vi "启动参数设置.vi"() -> ()   [LabVIEW 2016, in "斯坦道总磷总氮.lvlib"]
uses:
  <vilib>/Utility/miscctls.llb/LVPointTypeDef.ctl
  Listbox/Implementations/Listbox/Listbox.lvclass
  <vilib>/Utility/miscctls.llb/LVStringsAndValuesArrayTypeDef_U16.ctl
  Listbox/Implementations/Listbox Item/Listbox Item.lvclass
  Listbox/Implementations/Listbox/Listbox.lvclass/Listbox.ctl
  Listbox/Implementations/Listbox Item/Listbox Item.lvclass/Listbox Item.ctl
  <vilib>/Utility/config.llb/NI_LVConfig.lvlib
panel:
  in  "Move to Left":bool
  in  "Move to Right":bool
  in  "启用的参数":i32(listbox)
  in  "参数列表":i32(listbox)
  in  "取消":bool
  in  "确认":bool
  # "请选择启动参数"
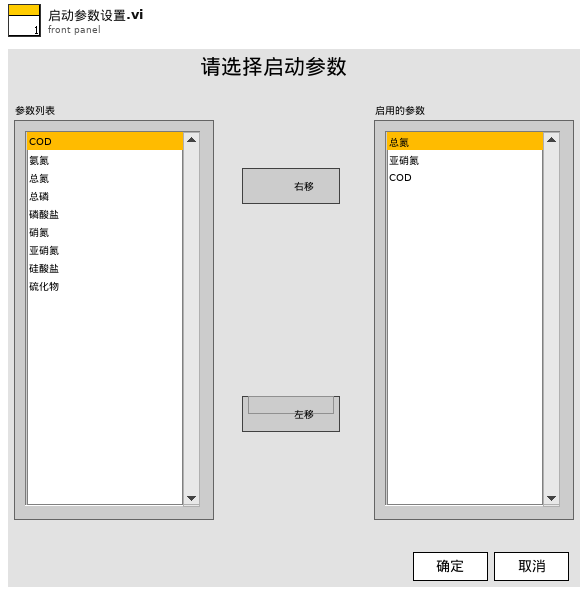
[diagram p1: front panel]
types:
  T1 = typedef "LVStringsAndValuesArrayTypeDef_U16.ctl" = cluster{"String":string, "Value":u16}[]
  T2 = typedef "LVPointTypeDef.ctl" = cluster{"Horizontal":i16, "Vertical":i16}
  T3 = typedef "NI_LVConfig.lvlib/Config Data RefNum.ctl" = refnum<k1>
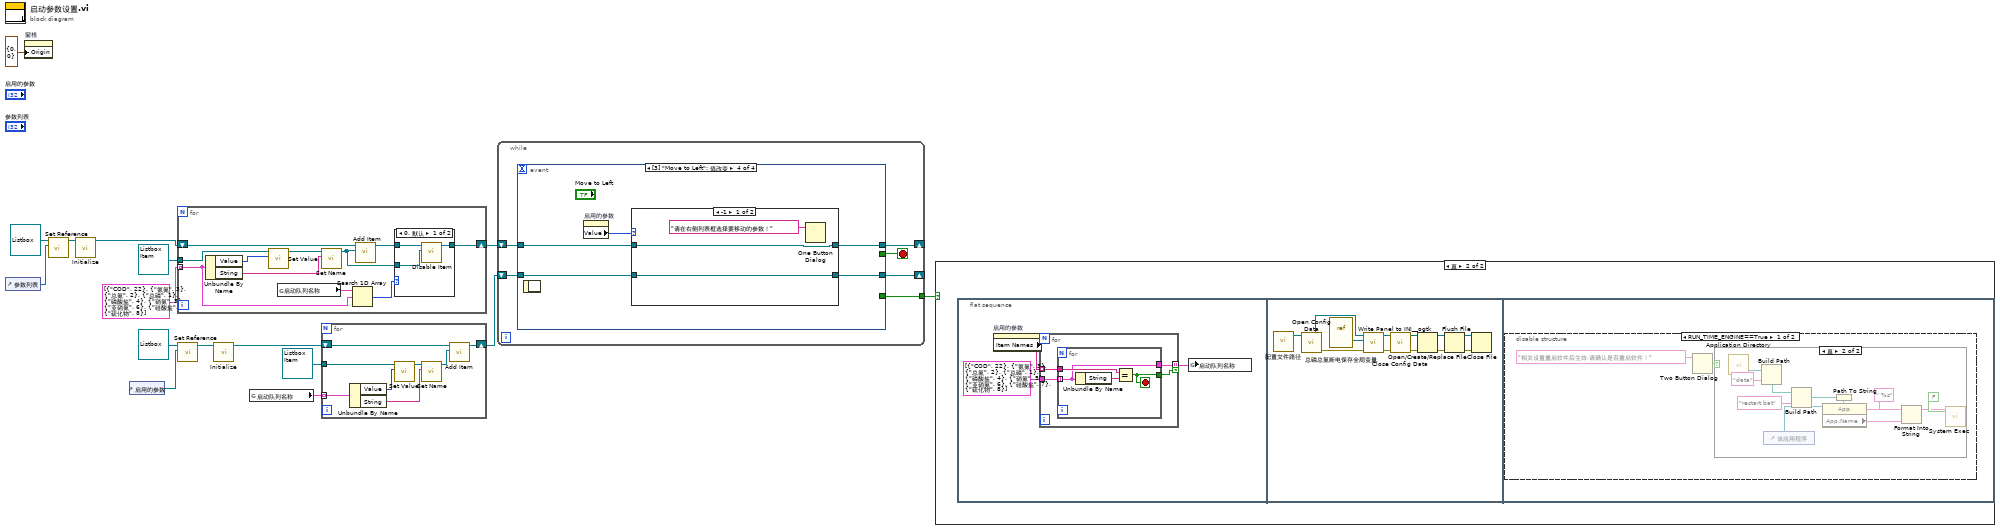
[diagram p0: block diagram]
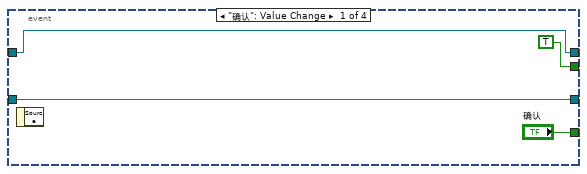
[diagram p2: hidden frame]
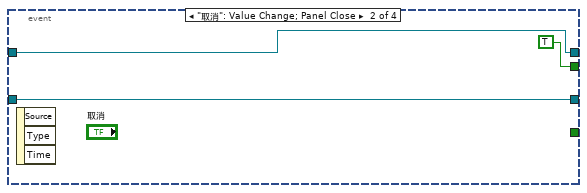
[diagram p3: hidden frame]
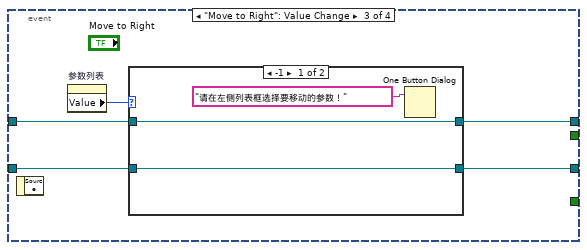
[diagram p4: hidden frame]
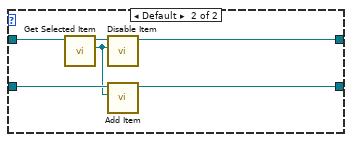
[diagram p5: hidden frame]
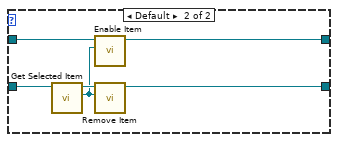
[diagram p6: hidden frame]
diagram:
  n1 = control-ref of="参数列表"() -> (w14:refnum<vi>)
  n2 = property on="窗格" class="Pane"("Origin"=T2 {"Horizontal"=0, "Vertical"=0} ("原点")) -> ()  [unwired: 2 in, 2 out]
  n3 = call "Set Reference.vi"("Reference"=w14, "Listbox in"=refnum<class "Listbox.lvclass"> refnum ("Listbox.lvclass")) -> ("Listbox out"=w13:refnum<class "Listbox.lvclass">)  [unwired: 9 in]
  n4 = call-dynamic "Initialize.vi"("Listbox in"=w13) -> ("Listbox out"=w10:refnum<class "Listbox.lvclass">)  [unwired: 9 in, 1 out]
  n5 = control-ref of="启用的参数"() -> (w11:refnum<vi>)
  n6 = for {
    tunnel: refnum<class "Listbox Item.lvclass"> refnum ("Listbox Item.lvclass") -> [w26]
    shift-right: [w18] -> w6
    shift-left: w10 -> [w27]
    tunnel: T1 [{"String"="COD", "Value"=22}, {"String"="氨氮", "Value"=3}, {"String"="总氮", "Value"=2}, {"String"="总磷", "Value"=1}, {"String"="磷酸盐", "Value"=4}, {"String"="硝氮", "Value"=5}, {"String"="亚硝氮", "Value"=6}, {"String"="硅酸盐", "Value"=7}, {"String"="硫化物", "Value"=8}] ("字符串与值[]") -> [w20] mode=indexing
    n7 = Unbundle By Name(w20) -> ("Value"=w23:u16, "String"=w24:string)
    n8 = call "Set Value.vi"("Value"=w23, "Listbox Item in"=w26) -> ("Listbox Item out"=w25:refnum<class "Listbox Item.lvclass">)  [unwired: 9 in]
    n9 = global read "总磷总氮断电保存全局变量.vi" "启动队列名称"() -> (w17:cluster{"String":string, "Value":u16}[])
    n10 = call "Set Name.vi"("Name"=w24, "Listbox Item in"=w25) -> ("Listbox Item out"=w21:refnum<class "Listbox Item.lvclass">)  [unwired: 9 in]
    n11 = Search 1D Array(1D array=w17, element=w20) -> (index of element=w19:i32)  [unwired: 1 in]
    n12 = call-dynamic "Add Item.vi"("Item"=w21, "Listbox in"=w27) -> ("Listbox out"=w22:refnum<class "Listbox.lvclass">)  [unwired: 8 in, 1 out]
    n13 = case shown="0, 默认" w19 {
      tunnel: w22 -> [w30 w31]
      tunnel: w21 -> [w29 _]
      tunnel: [w28 w31] -> w18
      frame 0, Default {
        n14 = call-dynamic "Disable Item.vi"("Item"=w29, "Listbox in"=w30) -> ("Listbox out"=w28:refnum<class "Listbox.lvclass">)  [unwired: 8 in, 1 out]
      }
      frame -1 {
      }
    }
  }
  n15 = call "Set Reference.vi"("Reference"=w11, "Listbox in"=refnum<class "Listbox.lvclass"> refnum ("Listbox.lvclass")) -> ("Listbox out"=w9:refnum<class "Listbox.lvclass">)  [unwired: 9 in]
  n16 = call-dynamic "Initialize.vi"("Listbox in"=w9) -> ("Listbox out"=w4:refnum<class "Listbox.lvclass">)  [unwired: 9 in, 1 out]
  n17 = global read "总磷总氮断电保存全局变量.vi" "启动队列名称"() -> (w1:cluster{"String":string, "Value":u16}[])
  n18 = for {
    tunnel: refnum<class "Listbox Item.lvclass"> refnum ("Listbox Item.lvclass") -> [w38]
    shift-right: [w32] -> w3
    shift-left: w4 -> [w39]
    tunnel: w1 -> [w33] mode=indexing
    n19 = Unbundle By Name(w33) -> ("Value"=w35:u16, "String"=w36:string)
    n20 = call "Set Value.vi"("Value"=w35, "Listbox Item in"=w38) -> ("Listbox Item out"=w37:refnum<class "Listbox Item.lvclass">)  [unwired: 9 in]
    n21 = call "Set Name.vi"("Name"=w36, "Listbox Item in"=w37) -> ("Listbox Item out"=w34:refnum<class "Listbox Item.lvclass">)  [unwired: 9 in]
    n22 = call-dynamic "Add Item.vi"("Item"=w34, "Listbox in"=w39) -> ("Listbox out"=w32:refnum<class "Listbox.lvclass">)  [unwired: 8 in, 1 out]
  }
  n23 = while {
    shift-right: [w43] -> _
    shift-left: w3 -> [w45]
    shift-right: [w42] -> _
    shift-left: w6 -> [w44]
    tunnel: [w40] -> w2
    stop <- w41 stop-if-true
    n24 = event shown="[3] \"Move to Left\": 值改变" {
      selector: _ -> [_ _ _ _]
      dyn-events: _ -> [_ _ _ _]
      timeout: _ -> [_ _ _ _]
      tunnel: w45 -> [w49 w52 w56 w71]
      tunnel: w44 -> [w48 w51 w57 w70]
      tunnel: [w49 w52 w54 w69] -> w43
      tunnel: [w48 w51 w55 w68] -> w42
      tunnel: [TRUE TRUE _ _] -> w41
      tunnel: ["确认" _ _ _] -> w40
      event "确认": Value Change {
        n25 = event-data() -> ()  [unwired: 1 in, 1 out]
      }
      event "取消": Value Change; Panel Close {
        n26 = event-data() -> ()  [unwired: 1 in, 3 out]
      }
      event "Move to Right": Value Change {
        n27 = event-data() -> ()  [unwired: 1 in, 1 out]
        n28 = property on="参数列表" class="LstBox (严格)"() -> ("Value"=w53:i32)  [unwired: 2 in, 2 out]
        n29 = case shown="-1" w53 {
          tunnel: w57 -> [w59 w66]
          tunnel: w56 -> [w60 w65]
          tunnel: [w59 w63] -> w55
          tunnel: [w60 w62] -> w54
          frame -1 {
            n30 = One Button Dialog(message="请在左侧列表框选择要移动的参数！" ("消息")) -> ()  [unwired: 1 in, 1 out]
          }
          frame Default {
            n31 = call-dynamic "Get Selected Item.vi"("Listbox in"=w66) -> ("Item"=w61:refnum<class "Item.lvclass">, "Listbox out"=w64:refnum<class "Listbox.lvclass">)  [unwired: 8 in, 1 out]
            n32 = call-dynamic "Disable Item.vi"("Item"=w61, "Listbox in"=w64) -> ("Listbox out"=w63:refnum<class "Listbox.lvclass">)  [unwired: 8 in, 1 out]
            n33 = call-dynamic "Add Item.vi"("Item"=w61, "Listbox in"=w65) -> ("Listbox out"=w62:refnum<class "Listbox.lvclass">)  [unwired: 8 in, 1 out]
          }
        }
      }
      event "Move to Left": Value Change {
        n34 = event-data() -> ()  [unwired: 1 in, 1 out]
        n35 = property on="启用的参数" class="LstBox (严格)"() -> ("Value"=w67:i32)  [unwired: 2 in, 2 out]
        n36 = case shown="-1" w67 {
          tunnel: w71 -> [w73 w80]
          tunnel: w70 -> [w74 w79]
          tunnel: [w73 w77] -> w69
          tunnel: [w74 w75] -> w68
          frame -1 {
            n37 = One Button Dialog(message="请在右侧列表框选择要移动的参数！" ("消息")) -> ()  [unwired: 1 in, 1 out]
          }
          frame Default {
            n38 = call-dynamic "Get Selected Item.vi"("Listbox in"=w80) -> ("Item"=w76:refnum<class "Item.lvclass">, "Listbox out"=w78:refnum<class "Listbox.lvclass">)  [unwired: 8 in, 1 out]
            n39 = call-dynamic "Enable Item.vi"("Item"=w76, "Listbox in"=w79) -> ("Listbox out"=w75:refnum<class "Listbox.lvclass">)  [unwired: 8 in, 1 out]
            n40 = call-dynamic "Remove Item.vi"("Item"=w76, "Listbox in"=w78) -> ("Listbox out"=w77:refnum<class "Listbox.lvclass">)  [unwired: 8 in, 1 out]
          }
        }
      }
    }
  }
  n41 = case shown="真" w2 {
    frame False {
    }
    frame True {
      n42 = flat-sequence {
        frame #0 {
          n43 = property on="启用的参数" class="LstBox (严格)"() -> ("Item Names"=w82:string[])  [unwired: 2 in, 2 out]
          n44 = for {
            tunnel: T1 [{"String"="COD", "Value"=22}, {"String"="氨氮", "Value"=3}, {"String"="总氮", "Value"=2}, {"String"="总磷", "Value"=1}, {"String"="磷酸盐", "Value"=4}, {"String"="硝氮", "Value"=5}, {"String"="亚硝氮", "Value"=6}, {"String"="硅酸盐", "Value"=7}, {"String"="硫化物", "Value"=8}] ("字符串与值[]") -> [w86]
            tunnel: w82 -> [w87] mode=indexing
            tunnel: [w85] -> w81 mode=indexing if=w84
            n45 = for {
              tunnel: w87 -> [w91]
              tunnel: w86 -> [w89] mode=indexing
              tunnel: [w89] -> w85
              tunnel: [w88] -> w84
              stop <- w88 stop-if-true
              n46 = Unbundle By Name(w89) -> ("String"=w90:string)
              n47 = Equal?(x=w91, y=w90) -> (x = y?=w88:bool)
            }
          }
          n48 = global write "总磷总氮断电保存全局变量.vi" "启动队列名称"(w81) -> ()
        }
        frame #1 {
          n49 = call "配置文件路径.vi"() -> ("appended path"=w92:path)  [unwired: 11 in]
          n50 = call <vilib>:"Open Config Data.vi"("configuration file path"=w92) -> ("error out"=w100:errorcluster, "refnum"=w103:T3)  [unwired: 8 in, 1 out]
          n51 = vi-ref "总磷总氮断电保存全局变量.vi"() -> (w102:refnum<vi>)
          n52 = call <userlib>:"Write Panel to INI__ogtk.vi"("error in (no error)"=w100, "VI ref"=w102, "refnum"=w103) -> ("error out"=w99:errorcluster, "refnum out"=w101:T3)  [unwired: 7 in]
          n53 = call <vilib>:"Close Config Data.vi"("error in (no error)"=w99, "refnum"=w101) -> ("error out"=w94:errorcluster, "file path"=w93:path)  [unwired: 8 in]
          n54 = Open/Create/Replace File(file path (use dialog)=w93, error in=w94) -> (refnum out=w97:refnum<file>, error out=w98:errorcluster)  [unwired: 4 in, 1 out]
          n55 = Flush File(refnum=w97, error in=w98) -> (refnum out=w96:refnum<file>, error out=w95:errorcluster)
          n56 = Close File(refnum=w96, error in=w95) -> ()  [unwired: 2 out]
        }
        frame #2 {
          n57 = disable-structure shown="RUN_TIME_ENGINE==True" {
            frame condition #0 {
              n58 = Two Button Dialog(message="相关设置重启软件后生效,请确认是否重启软件！" ("按钮名称（“确定”）")) -> (T button?=w105:bool)  [unwired: 2 in]
              n59 = case shown="真" w105 {
                frame False {
                }
                frame True {
                  n60 = call <vilib>:"Application Directory.vi"() -> ("Application Directory"=w107:path)
                  n61 = Build Path(base path=w107, name or relative path="data" ("名称或相对路径")) -> (appended path=w109:path)
                  n62 = control-ref of="该应用程序"() -> (w106:refnum<vi>)
                  n63 = Build Path(base path=w109, name or relative path="restart.bat" ("名称或相对路径")) -> (appended path=w111:path)
                  n64 = property class="App"(reference=w106) -> ("App.Name"=w114:string)  [unwired: 1 in, 2 out]
                  n65 = Path To String(path=w111) -> (string=w112:string)
                  n66 = Format Into String(format string=" %s" ("格式字符串"), initial string=w112, w114) -> (resulting string=w115:string)  [unwired: 1 in, 1 out]
                  n67 = call <vilib>:"System Exec.vi"("wait until completion? (T)"=FALSE, "command line"=w115) -> ()  [unwired: 6 in, 4 out]
                }
              }
            }
            frame condition #1 (active) {
            }
          }
        }
      }
    }
  }
